vi "Rotate Array_U32.vi"(9 "Clockwise":bool caption="CounterClockwise", 11 "Array":u32[][](array[numeric])) -> (3 "Rotated Array":u32[][](array[numeric]))   [LabVIEW 2020]
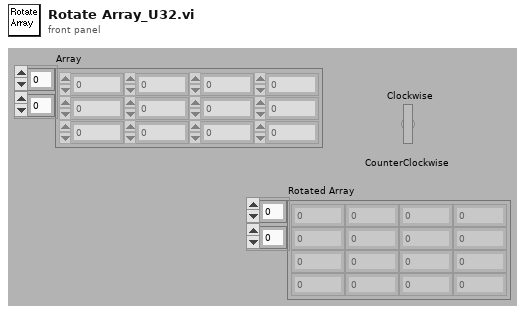
[diagram p1: front panel]
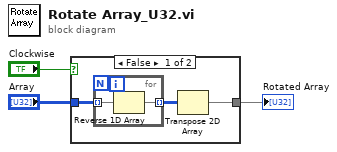
[diagram p0: block diagram]
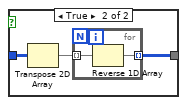
[diagram p2: hidden frame]
diagram:
  n1 = case shown="False" "Clockwise" {
    tunnel: "Array" -> [w6 w11]
    tunnel: [w4 w9] -> w1
    frame False {
      n2 = for {
        tunnel: [w8] -> w5 mode=indexing
        tunnel: w6 -> [w7] mode=indexing
        n3 = Reverse 1D Array(array=w7) -> (reversed array=w8:u32[])
      }
      n4 = Transpose 2D Array(2D array=w5) -> (transposed array=w4:u32[][])
    }
    frame True {
      n5 = Transpose 2D Array(2D array=w11) -> (transposed array=w10:u32[][])
      n6 = for {
        tunnel: [w13] -> w9 mode=indexing
        tunnel: w10 -> [w12] mode=indexing
        n7 = Reverse 1D Array(array=w12) -> (reversed array=w13:u32[])
      }
    }
  }
  "Rotated Array" <- w1
